vi "Evaluate.vi"(8 "error in (no error)":errorcluster, 11 "Never In":refnum<class "Never.lvclass">) -> (0 "error out":errorcluster, 1 "Message":string, 2 "Passed?":bool)   [LabVIEW 2020, in "Never.lvlib" / "Never.lvclass"]
uses:
  Never.lvclass
  Never.lvclass/Never.ctl
  Core/VI Call/VI Call.lvclass
  Core/Comparator/Comparator.lvclass
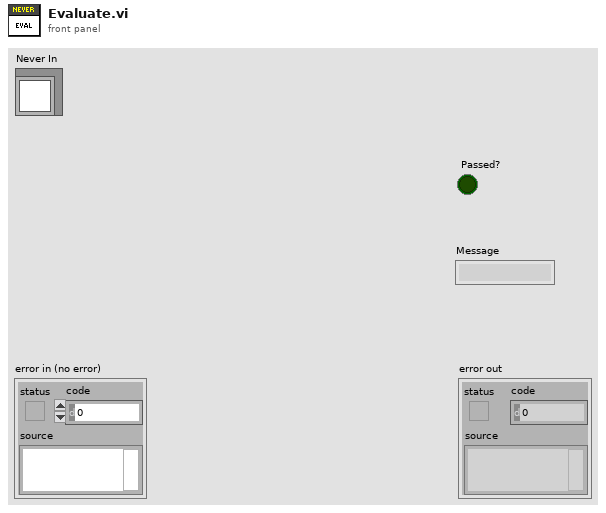
[diagram p1: front panel]
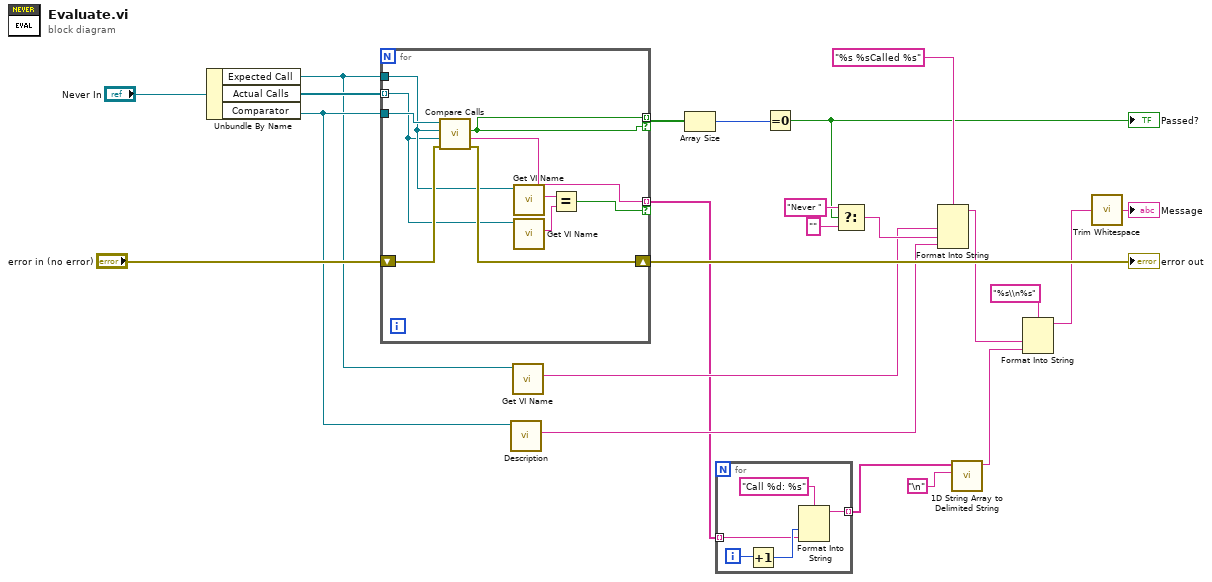
[diagram p0: block diagram]
diagram:
  n1 = Unbundle By Name("Never In") -> ("Expected Call"=w10:refnum<class "VI Call.lvclass">, "Actual Calls"=w21:refnum<class "VI Call.lvclass">[], "Comparator"=w12:refnum<class "Comparator.lvclass">)
  n2 = for {
    tunnel: w10 -> [w25]
    tunnel: w12 -> [w33]
    tunnel: w21 -> [w24] mode=indexing
    shift-right: [w31] -> w20
    shift-left: "error in (no error)" -> [w32]
    tunnel: [w30] -> w19 mode=indexing if=w30
    tunnel: [w27] -> w2 mode=indexing if=w26
    n3 = call-dynamic "Compare Calls.vi"("error in (no error)"=w32, "VI Call 2"=w24, "VI Call 1"=w25, "Comparator in"=w33) -> ("error out"=w31:errorcluster, "Description"=w27:string, "Equal?"=w30:bool)  [unwired: 5 in]
    n4 = call-dynamic "Get VI Name.vi"("VI Call In"=w25) -> ("VI Name"=w28:string)  [unwired: 9 in, 1 out]
    n5 = call-dynamic "Get VI Name.vi"("VI Call In"=w24) -> ("VI Name"=w29:string)  [unwired: 9 in, 1 out]
    n6 = Equal?(x=w28, y=w29) -> (x = y?=w26:bool)
  }
  "error out" <- w20
  n7 = call-dynamic "Description.vi"("Comparator in"=w12) -> ("Description"=w11:string)  [unwired: 9 in, 1 out]
  n8 = call-dynamic "Get VI Name.vi"("VI Call In"=w10) -> ("VI Name"=w9:string)  [unwired: 9 in, 1 out]
  n9 = Array Size(array=w19) -> (size(s)=w18:i32)
  n10 = for {
    tunnel: w2 -> [w35] mode=indexing
    tunnel: [w34] -> w1 mode=indexing
    i -> [w37]
    n11 = Increment(x=w37) -> (x+1=w36:i32)
    n12 = Format Into String(format string="Call %d: %s", w36, w35) -> (resulting string=w34:string)  [unwired: 2 in, 1 out]
  }
  n13 = Equal To 0?(x=w18) -> (x = 0?=w13:bool)
  "Passed?" <- w13
  n14 = Select(t="Never ", s=w13, f="") -> (s? t:f=w15:string)
  n15 = Format Into String(format string="%s %sCalled %s" ("Message"), w9, w15, w11) -> (resulting string=w5:string)  [unwired: 2 in, 1 out]
  n16 = call <vilib>:"1D String Array to Delimited String.vi"("delimiter"="\n", "string array"=w1) -> ("delimited string"=w4:string)  [unwired: 9 in]
  n17 = Format Into String(format string="%s\\n%s", w5, w4) -> (resulting string=w6:string)  [unwired: 2 in, 1 out]
  n18 = call <vilib>:"Trim Whitespace.vi"("string"=w6) -> ("trimmed string"=→"Message":string)  [unwired: 1 in]
